vi "Calibrate DSA AO With DMM.vi"(7 "DAQ output range":dbl=5.0, 8 "error in":errorcluster, 11 "device sessions":T2) -> (0 "error out":errorcluster, 1 "Calibration done":bool, 2 "intercept":dbl, 3 "slope":dbl)   [LabVIEW 2021, in "Full Scale Error_ADC.lvlib"]
uses:
  Full Scale Error_ADC.lvlib
  <vilib>/gRPC/LabVIEW gRPC Library/Shared/grpcId.ctl
  <instrlib>/niDMM/nidmm.llb/niDMM Resolution in Digits.ctl
  <instrlib>/niDMM/nidmm.llb/niDMM Function.ctl
  <vilib>/DAQmx/write.llb/DAQmx Write (Analog 1D DBL 1Chan NSamp).vi
  <instrlib>/niDMM/nidmm.llb/niDMM Configure Measurement Digits.vi
  <vilib>/DAQmx/miscellaneous.llb/DAQmx Fill In Error Info.vi
  <vilib>/Analysis/NI_AALPro.lvlib
  <vilib>/gRPC/LabVIEW gRPC Library/grpc-lvsupport-release.lvlib
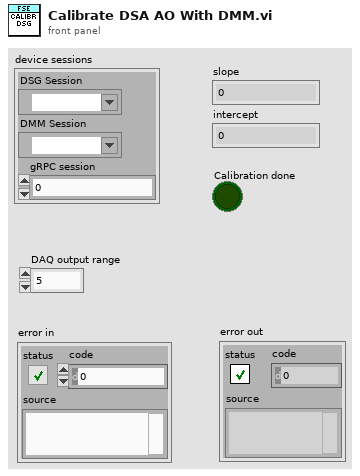
[diagram p1: front panel]
types:
  T1 = typedef "grpc-lvsupport-release.lvlib/grpcId.ctl" = u64
  T2 = cluster{"DSG Session":refnum<k21>, "DMM Session":refnum<k15>, "gRPC session":T1}
  T3 = typedef "niDMM Function.ctl" = enum16{"DC Volts", "AC Volts", "DC Current", "AC Current", "2-wire Resistance", "4-wire Resistance", "Diode", "Frequency", "Period", "AC Volts DC Coupled", "Capacitance", "Inductance", "Temperature"}
  T4 = typedef "niDMM Resolution in Digits.ctl" = dbl
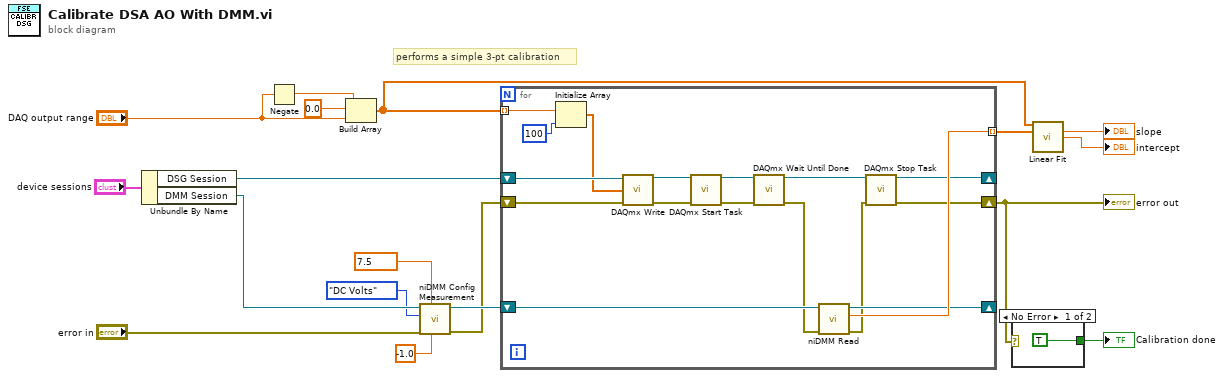
[diagram p0: block diagram]
diagram:
  w10 = T4 7.5 items=["3 1/2"=3.5, "4 1/2"=4.5, "5 1/2"=5.5, "6 1/2"=6.5, "7 1/2"=7.5] ("Resolution in Digits")
  # "performs a simple 3-pt calibration"
  n1 = Unbundle By Name("device sessions") -> ("DSG Session"=w15:refnum<k21>, "DMM Session"=w14:refnum<k15>)
  n2 = Negate(x="DAQ output range") -> (-x=w5:dbl)
  n3 = Build Array(w5, 0.0 ("element"), "DAQ output range") -> (w3:dbl[])
  n4 = call-poly <instrlib>:"niDMM Config Measurement.vi"("Range"=-1.0, "Resolution in Digits"=w10, "error in (no error)"="error in", "Function"=niDMM_Function."DC Volts" ("Measurement Type"), "instrument handle"=w14) -> ("error out"=w7:errorcluster, "instrument handle out"=w8:refnum<k15>)  [unwired: 5 in]
  n5 = for {
    tunnel: w3 -> [w26] mode=indexing
    shift-right: [w19] -> w18
    shift-left: w7 -> [w25]
    tunnel: [w24] -> w6 mode=indexing
    shift-right: [w23] -> _
    shift-left: w15 -> [w30]
    shift-right: [w22] -> _
    shift-left: w8 -> [w27]
    n6 = Initialize Array(w26, 100 ("dimension size")) -> (w29:dbl[])
    n7 = call-poly <vilib>:"DAQmx Write.vi"("task/channels in"=w30, "data"=w29, "error in"=w25) -> ("task out"=w32:refnum<k21>, "error out"=w31:errorcluster)  [unwired: 10 in, 1 out]
    n8 = call <vilib>:"DAQmx Start Task.vi"("task/channels in"=w32, "error in"=w31) -> ("task out"=w35:refnum<k21>, "error out"=w34:errorcluster)  [unwired: 12 in]
    n9 = call <vilib>:"DAQmx Wait Until Done.vi"("task/channels in"=w35, "error in"=w34) -> ("task out"=w33:refnum<k21>, "error out"=w21:errorcluster)  [unwired: 12 in]
    n10 = call <instrlib>:"niDMM Read.vi"("error in (no error)"=w21, "instrument handle"=w27) -> ("error out"=w20:errorcluster, "Measurement"=w24:dbl, "instrument handle out"=w22:refnum<k15>)  [unwired: 7 in]
    n11 = call <vilib>:"DAQmx Stop Task.vi"("task/channels in"=w33, "error in"=w20) -> ("task out"=w23:refnum<k21>, "error out"=w19:errorcluster)  [unwired: 12 in]
  }
  "error out" <- w18
  n12 = case shown="No Error" w18 {
    tunnel: [TRUE _] -> w2
    frame No Error {
    }
    frame Error {
    }
  }
  "Calibration done" <- w2
  n13 = call <vilib>:"Linear Fit.vi"("Y"=w3, "X"=w6) -> ("slope"=→"slope":dbl, "intercept"=→"intercept":dbl)  [unwired: 9 in, 3 out]
